vi "23384_Davis_Poku_Amankwa_Amankwa.DavisPoku.MNE1201.8.1_348265_2062580935.vi"() -> ()   [LabVIEW 2018]
panel:
  in  "stop":bool
  out "1":bool
  out "4":bool
  out "3":bool
  out "2":bool
  out "0":bool
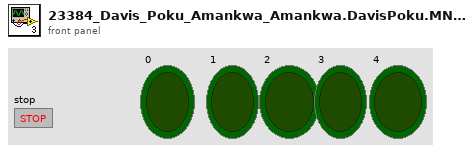
[diagram p1: front panel]
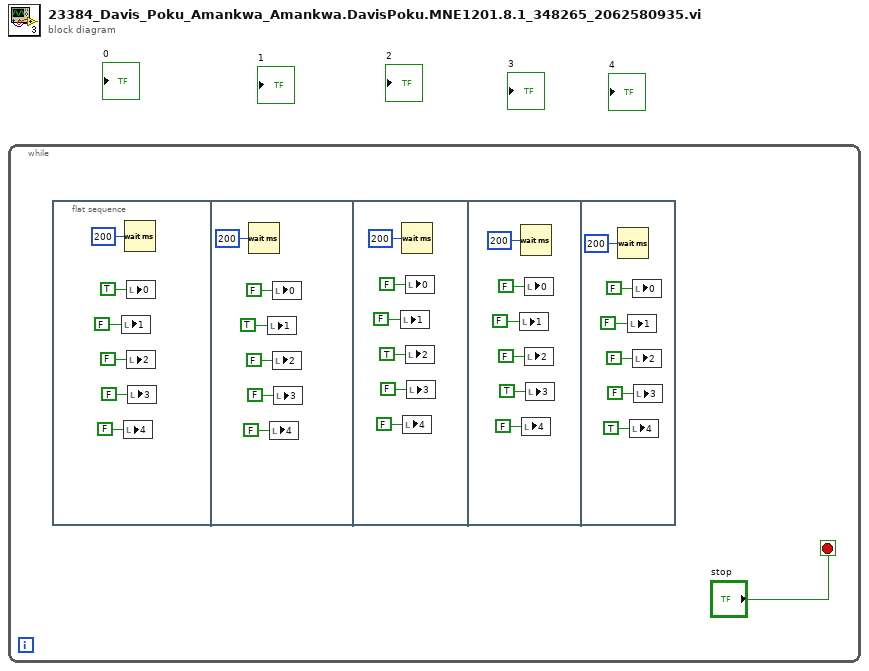
[diagram p0: block diagram]
diagram:
  n1 = while {
    stop <- "stop" stop-if-true
    n2 = flat-sequence {
      frame #0 {
        n3 = local write "1"(FALSE) -> ()
        n4 = local write "4"(FALSE) -> ()
        n5 = Wait (ms)(milliseconds to wait=u32 200) -> ()  [unwired: 1 out]
        n6 = local write "0"(TRUE) -> ()
        n7 = local write "2"(FALSE) -> ()
        n8 = local write "3"(FALSE) -> ()
      }
      frame #1 {
        n9 = Wait (ms)(milliseconds to wait=u32 200) -> ()  [unwired: 1 out]
        n10 = local write "1"(TRUE) -> ()
        n11 = local write "4"(FALSE) -> ()
        n12 = local write "0"(FALSE) -> ()
        n13 = local write "2"(FALSE) -> ()
        n14 = local write "3"(FALSE) -> ()
      }
      frame #2 {
        n15 = local write "1"(FALSE) -> ()
        n16 = Wait (ms)(milliseconds to wait=u32 200) -> ()  [unwired: 1 out]
        n17 = local write "4"(FALSE) -> ()
        n18 = local write "0"(FALSE) -> ()
        n19 = local write "2"(TRUE) -> ()
        n20 = local write "3"(FALSE) -> ()
      }
      frame #3 {
        n21 = local write "1"(FALSE) -> ()
        n22 = Wait (ms)(milliseconds to wait=u32 200) -> ()  [unwired: 1 out]
        n23 = local write "4"(FALSE) -> ()
        n24 = local write "0"(FALSE) -> ()
        n25 = local write "2"(FALSE) -> ()
        n26 = local write "3"(TRUE) -> ()
      }
      frame #4 {
        n27 = Wait (ms)(milliseconds to wait=u32 200) -> ()  [unwired: 1 out]
        n28 = local write "1"(FALSE) -> ()
        n29 = local write "4"(TRUE) -> ()
        n30 = local write "0"(FALSE) -> ()
        n31 = local write "2"(FALSE) -> ()
        n32 = local write "3"(FALSE) -> ()
      }
    }
  }
